vi "Main_12b.vi"() -> ()   [LabVIEW 2020]
uses:
  Cluster Point.ctl
panel:
  out "size":i32
  out "Array 3":i32[](array[numeric])
  out "itt":i32
  out "enpoint value":i32
  out "Array 2":i32[][](array[numeric])
  out "Map":map{T1, i32}(c390)
  out "Array":u8[][](array[numeric])
  out "End":T1
  out "Start":T1
  out "Answer":i32
  in  "Puzzle":string="abcccccccccccccccccccccccccccccccaaaaaaaaaaaaaaaaccaaaaaaaaccccccccccccccccccccccccccccccccccccaaaaaa\nabcccccccccccccccccccccccccccccccaaaaaaaaaaaaaaaaaccaaaaaaccccccccccccccccccccccccccccccccccccccaaaaa\nabcccccccccccccccccccccccccccccccccaaaaaaaacccaaaaccaaaaaaccccccccccccccccccccaaaccccccccccccccccaaaa\nabcccccccccccccccccccccccccccccccccccaaaaaaaccaaccccaaaaaaccccccccccccccccccccaaaccccccccccccccccaaaa\nabcccccccccccccccccccccccccccccaaacccaaaaaaaacccccccaaccaaccccccccccccccccccccaaaccccccccccccccccaaac\nabcccccccccccccccccccccccccccccaaaaaaaaacaaaacccccccccccccccaccaaccccccccccccciiaaccaaaccc..."
  in  "Example":string="Sabqponm\nabcryxxl\naccszExk\nacctuvwj\nabdefghi"
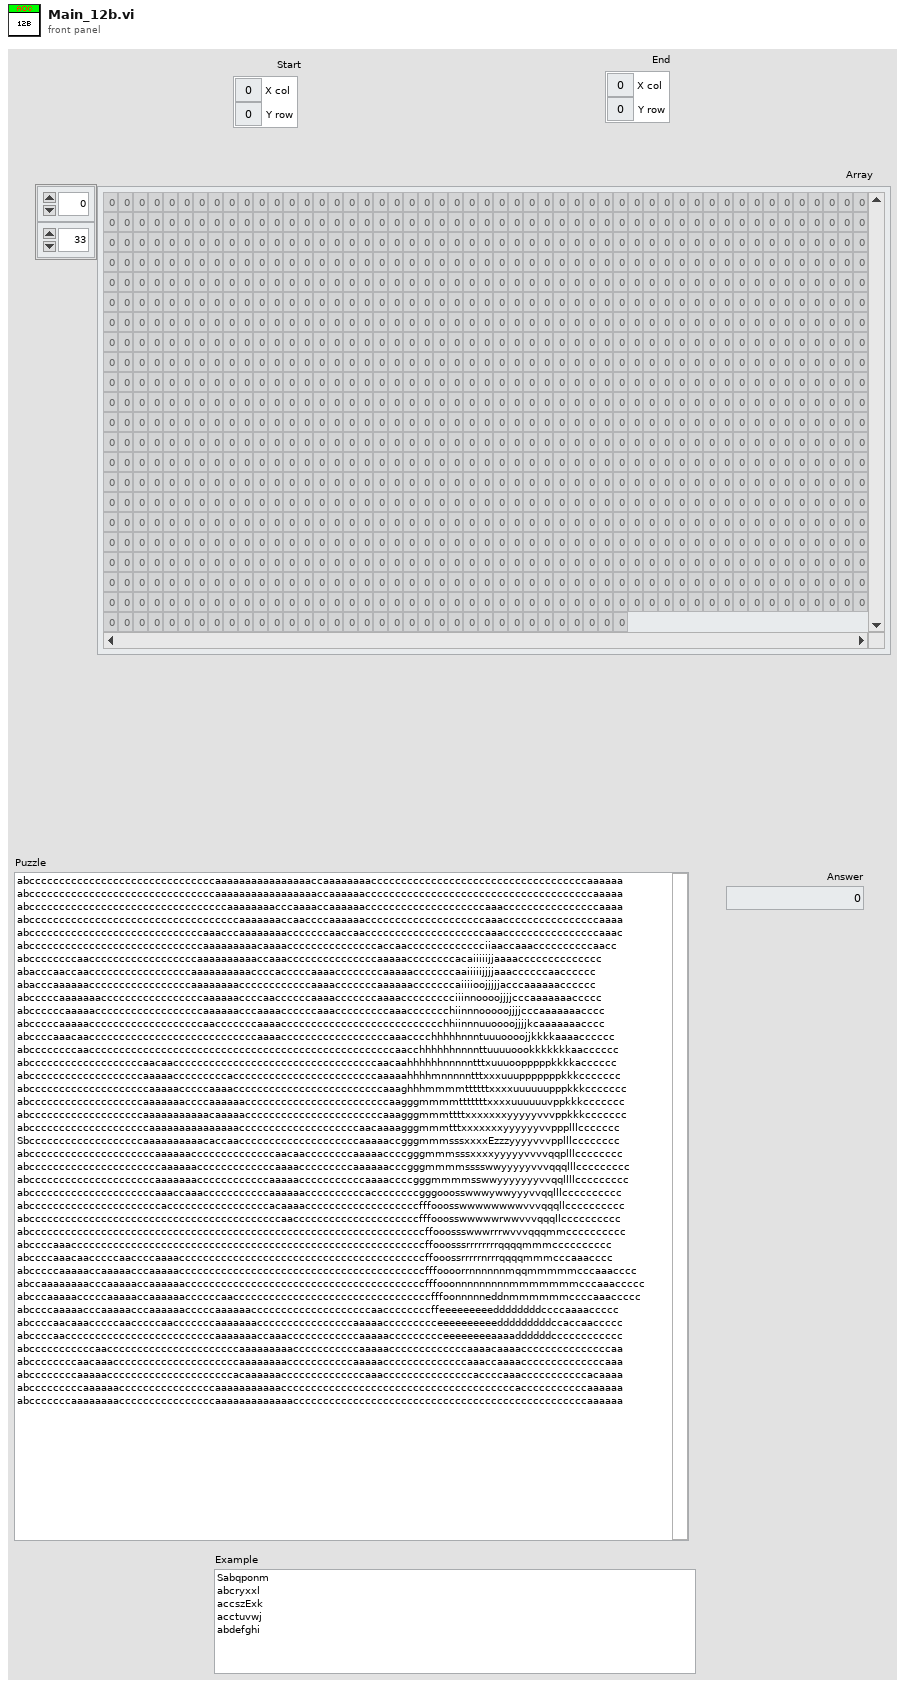
[diagram p1: front panel]
types:
  T1 = typedef "Cluster Point.ctl" = cluster{"X col":i32, "Y row":i32}
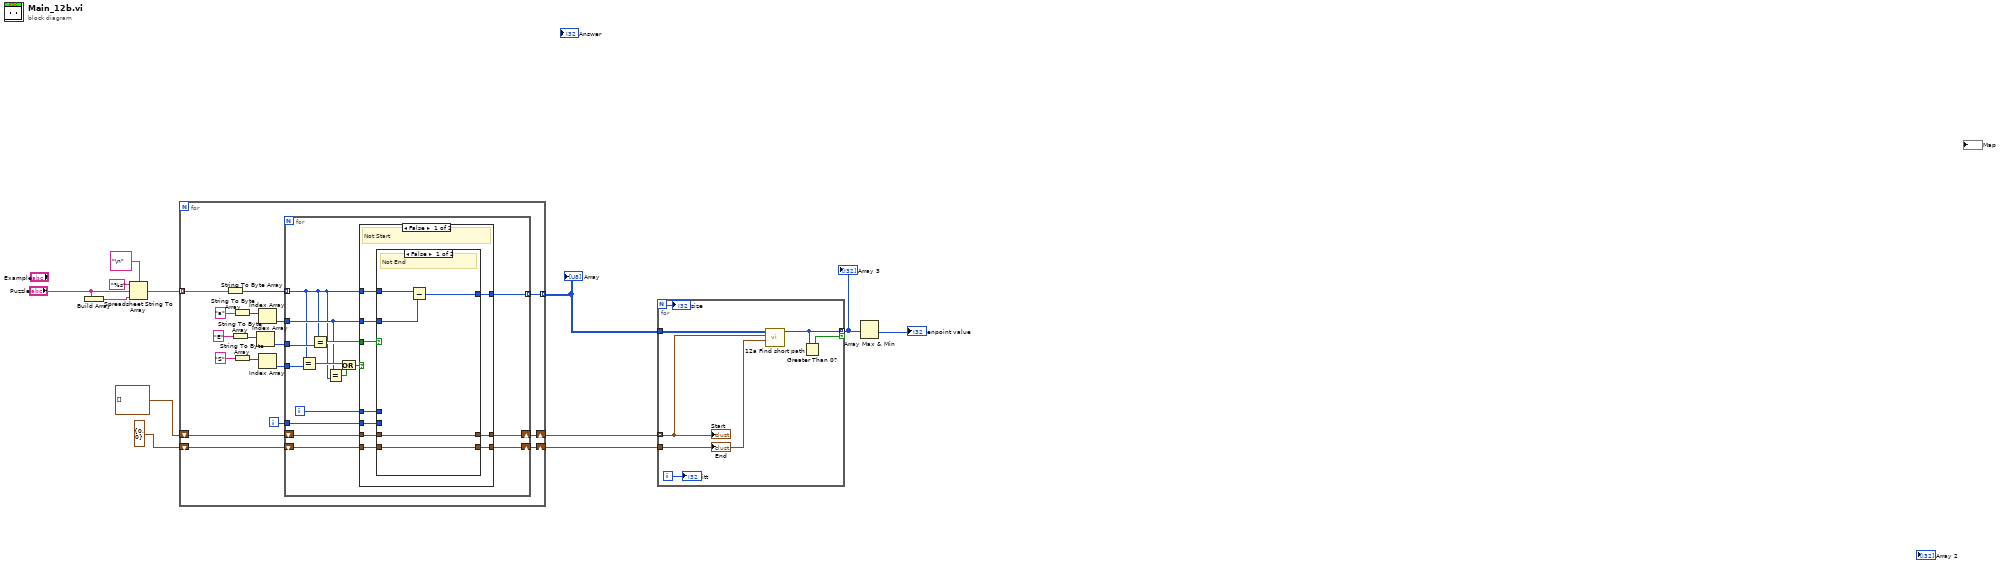
[diagram p0: block diagram]
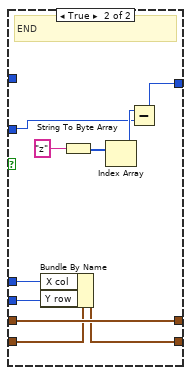
[diagram p2: hidden frame]
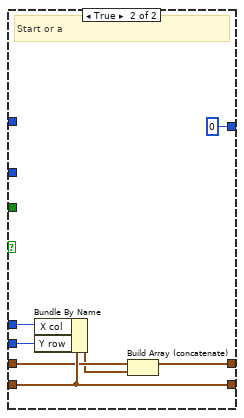
[diagram p3: hidden frame]
diagram:
  n1 = Build Array("Puzzle") -> (w12:string[])
  n2 = Spreadsheet String To Array(delimiter (Tab)="\n", format string="%s", spreadsheet string="Puzzle", array type (2D Dbl)=w12) -> (array=w9:string[])
  n3 = for {
    tunnel: w9 -> [w29] mode=indexing
    shift-right: [w14] -> w6
    shift-left: T1[] [] ("Array") -> [w18]
    shift-right: [w13] -> w5
    shift-left: T1 {"X col"=0, "Y row"=0} ("Point") -> [w17]
    tunnel: [w15] -> w7 mode=indexing
    i -> [w16]
    n4 = String To Byte Array(string=w29) -> (unsigned byte array=w26:u8[])
    n5 = String To Byte Array(string="E") -> (unsigned byte array=w24:u8[])
    n6 = String To Byte Array(string="a") -> (unsigned byte array=w27:u8[])
    n7 = String To Byte Array(string="S") -> (unsigned byte array=w21:u8[])
    n8 = Index Array(array=w24) -> (element=w20:u8)  [unwired: 1 in]
    n9 = Index Array(array=w27) -> (element=w25:u8)  [unwired: 1 in]
    n10 = Index Array(array=w21) -> (element=w19:u8)  [unwired: 1 in]
    n11 = for {
      tunnel: w26 -> [w32] mode=indexing
      tunnel: w25 -> [w33]
      tunnel: w20 -> [w44]
      tunnel: w19 -> [w43]
      shift-right: [w38] -> w14
      shift-left: w18 -> [w37]
      shift-right: [w35] -> w13
      shift-left: w17 -> [w36]
      tunnel: w16 -> [w39]
      tunnel: [w34] -> w15 mode=indexing
      i -> [w40]
      n12 = Equal?(x=w32, y=w43) -> (x = y?=w42:bool)
      n13 = Equal?(x=w32, y=w44) -> (x = y?=w41:bool)
      n14 = Equal?(x=w33, y=w32) -> (x = y?=w30:bool)
      n15 = Or(x=w42, y=w30) -> (x .or. y?=w31:bool)
      n16 = case shown="False" w31 {
        tunnel: w32 -> [w53 _]
        tunnel: w41 -> [w54 _]
        tunnel: w40 -> [w51 w76]
        tunnel: w39 -> [w50 w75]
        tunnel: [w46 w70] -> w38
        tunnel: w37 -> [w48 w72]
        tunnel: w36 -> [w47 w73]
        tunnel: [w49 w73] -> w35
        tunnel: [w52 u8 0] -> w34
        tunnel: w33 -> [w45 _]
        frame False {
          # "Not Start"
          n17 = case shown="False" w54 {
            tunnel: w53 -> [w59 _]
            tunnel: [w57 w60] -> w52
            tunnel: w51 -> [_ w63]
            tunnel: w50 -> [_ w64]
            tunnel: [w55 w66] -> w49
            tunnel: w48 -> [w56 w67]
            tunnel: w47 -> [w55 w65]
            tunnel: [w56 w67] -> w46
            tunnel: w45 -> [w58 w61]
            frame False {
              # "Not End"
              n18 = Subtract(x=w59, y=w58) -> (x-y=w57:u8)
            }
            frame True {
              # "END"
              n19 = Bundle By Name(cluster=w65, "X col"=w63, "Y row"=w64) -> (w66:T1)
              n20 = String To Byte Array(string="z") -> (unsigned byte array=w68:u8[])
              n21 = Index Array(array=w68) -> (element=w62:u8)  [unwired: 1 in]
              n22 = Subtract(x=w62, y=w61) -> (x-y=w60:u8)
            }
          }
        }
        frame True {
          # "Start or a"
          n23 = Bundle By Name(cluster=w73, "X col"=w76, "Y row"=w75) -> (w71:T1)
          n24 = Build Array (concatenate)(w72, w71) -> (w70:T1[])
        }
      }
    }
  }
  "Array" <- w7
  n25 = for {
    N -> [w79]
    tunnel: w7 -> [w83]
    tunnel: [w78] -> w3 mode=indexing if=w77
    tunnel: w6 -> [w82] mode=indexing
    tunnel: w5 -> [w81]
    i -> [w80]
    n26 = call "12a Find short path.vi"("End Point>>"=w81, "Start Point"=w82, "Field Elevation"=w83) -> ("Enpoint Value Out"=w78:i32)  [unwired: 6 in, 2 out]
    n27 = Greater Than 0?(x=w78) -> (x > 0?=w77:bool)
    "Start" <- w82
    "End" <- w81
    "itt" <- w80
    "size" <- w79
  }
  "Array 3" <- w3
  n28 = Array Max & Min(array=w3) -> (min value=→"enpoint value":i32)  [unwired: 3 out]
